vi "LaserStatusDigInt.vi"(9 "21":bool, 10 "16":bool, 11 "11":bool) -> (1 "Laser Status":T1)   [LabVIEW 2014]
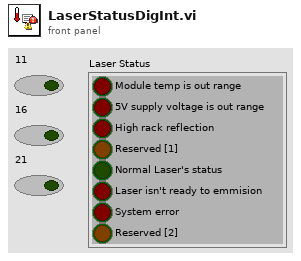
[diagram p1: front panel]
types:
  T1 = cluster{"Module temp is out range":bool, "5V supply voltage is out range":bool, "High rack reflection":bool, "Reserved [1]":bool, "Normal Laser's status":bool, "Laser isn't ready to emmision":bool, "System error":bool, "Reserved [2]":bool}
  T2 = cluster{"[0]":bool, "[1]":bool, "[2]":bool, "[3]":bool, "[4]":bool, "[5]":bool, "[6]":bool, "[7]":bool}
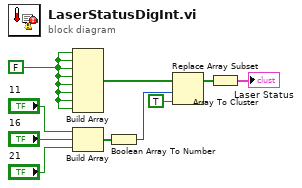
[diagram p0: block diagram]
diagram:
  w5 = FALSE ("element")
  n1 = Build Array(w5, w5, w5, w5, w5, w5, w5, w5) -> (w3:bool[])
  n2 = Build Array("11", "16", "21") -> (w8:bool[])
  n3 = Boolean Array To Number(Boolean array=w8) -> (number=w2:u32)
  n4 = Replace Array Subset(array=w3, new element=TRUE ("new element/subarray"), index=w2) -> (w4:bool[])
  n5 = Array To Cluster(array=w4) -> (cluster=→"Laser Status":T2)
